vi "Prepend +.vi"(1 "Input String":string) -> (0 "Space + Input String":string)   [LabVIEW 2020]
doc: "This VI inserts a space at the beginning of a string.\nScott Hannahs, FBNML, Jan 1992"
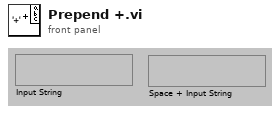
[diagram p1: front panel]
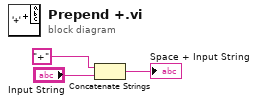
[diagram p0: block diagram]
diagram:
  n1 = Concatenate Strings("+", "Input String") -> (→"Space + Input String":string)
